vi "GetType.vi"(8 "error in (no error)":errorcluster, 11 "Quench Msg":refnum<class "Quench Msg.lvclass">) -> (0 "error out":errorcluster, 2 "Data Sample":variant, 3 "Quench Msg":refnum<class "Quench Msg.lvclass">)   [LabVIEW 2016, in "KIT-QVA.lvlib" / "Quench Msg.lvclass"]
doc: "This VI delivers a sample of the data type format the message expects."
uses:
  Quench Msg.lvclass
  Quench Msg.lvclass/Quench Msg.ctl
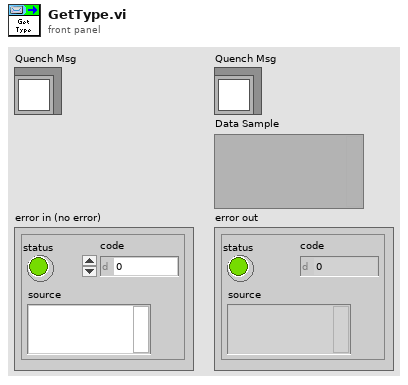
[diagram p1: front panel]
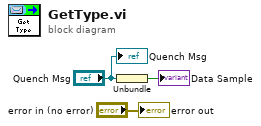
[diagram p0: block diagram]
diagram:
  n1 = Unbundle("Quench Msg") -> (→"Data Sample":bool)
  "error out" <- "error in (no error)"
  "Quench Msg" <- "Quench Msg"
